vi "xboxToggle.vi"   [LabVIEW 2017]
uses:
  globalUtilities.vi
types:
  T1 = cluster{"button info":cluster{"button 1":bool, "button 2":bool, "button 3":bool, "button 4":bool, "button 5":bool, "button 6":bool, "button 7":bool, "button 8":bool, "button 9":bool, "button 10":bool, "button 11":bool, "button 12":bool, "button 13":bool, "button 14":bool, "button 15":bool, "button 16":bool, "button 17":bool, "button 18":bool, "button 19":bool, "button 20":bool, "button 21":bool, "button 22":bool, "button 23":bool, "button 24":bool, "button 25":bool, "button 26":bool, "button 27":bool, "button 28":bool, "button 29":bool, "button 30":bool, "button 31":bool, "button 32":bool}, "direction info":cluster{"pov 1":i32, "pov 2":i32, "pov 3":i32, "pov 4":i32}, "axis info":cluster{"X axis":i32, "Y axis":i32, "Z axis":i32, "X axis rotation":i32, "Y axis rotation":i32, "Z axis rotation":i32, "U axis":i32, "V axis":i32}}
  T2 = cluster{"button 1":bool, "button 2":bool, "button 3":bool, "button 4":bool, "button 5":bool, "button 6":bool, "button 7":bool, "button 8":bool, "button 9":bool, "button 10":bool, "button 11":bool, "button 12":bool, "button 13":bool, "button 14":bool, "button 15":bool, "button 16":bool, "button 17":bool, "button 18":bool, "button 19":bool, "button 20":bool, "button 21":bool, "button 22":bool, "button 23":bool, "button 24":bool, "button 25":bool, "button 26":bool, "button 27":bool, "button 28":bool, "button 29":bool, "button 30":bool, "button 31":bool, "button 32":bool}
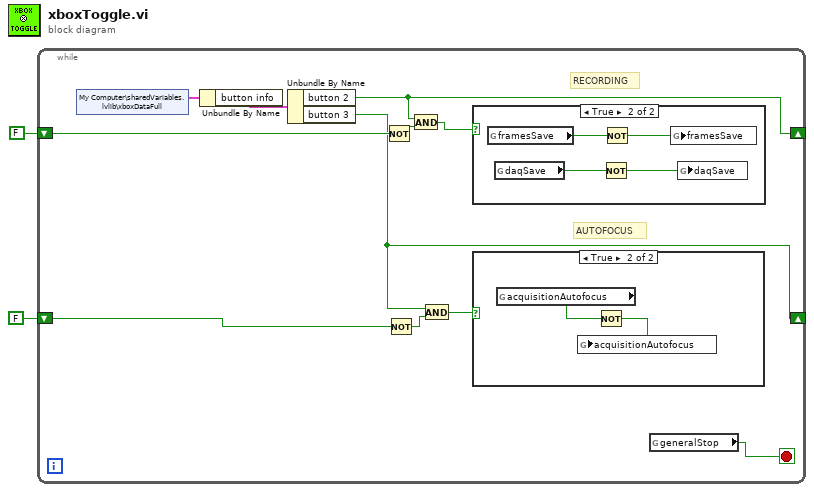
[diagram p0: block diagram]
diagram:
  n1 = while {
    shift-right: [w10] -> _
    shift-left: FALSE -> [w11]
    shift-right: [w3] -> _
    shift-left: FALSE -> [w6]
    stop <- w7 stop-if-true
    # "AUTOFOCUS"
    # "RECORDING"
    n2 = shared-variable "My Computer\\sharedVariables.lvlib\\xboxDataFull"() -> (w13:T1)  [unwired: 1 in, 1 out]
    n3 = Unbundle By Name(w13) -> ("button info"=w12:T2)
    n4 = Unbundle By Name(w12) -> ("button 2"=w10:bool, "button 3"=w3:bool)
    n5 = Not(x=w11) -> (.not. x?=w9:bool)
    n6 = Not(x=w6) -> (.not. x?=w5:bool)
    n7 = And(x=w10, y=w9) -> (x .and. y?=w8:bool)
    n8 = And(x=w3, y=w5) -> (x .and. y?=w4:bool)
    n9 = case shown="True" w8 {
      frame False {
      }
      frame True {
        n10 = global read "globalUtilities.vi" "framesSave"() -> (w19:bool)
        n11 = global read "globalUtilities.vi" "daqSave"() -> (w16:bool)
        n12 = Not(x=w16) -> (.not. x?=w17:bool)
        n13 = Not(x=w19) -> (.not. x?=w18:bool)
        n14 = global write "globalUtilities.vi" "framesSave"(w18) -> ()
        n15 = global write "globalUtilities.vi" "daqSave"(w17) -> ()
      }
    }
    n16 = case shown="True" w4 {
      frame False {
      }
      frame True {
        n17 = global read "globalUtilities.vi" "acquisitionAutofocus"() -> (w15:bool)
        n18 = Not(x=w15) -> (.not. x?=w14:bool)
        n19 = global write "globalUtilities.vi" "acquisitionAutofocus"(w14) -> ()
      }
    }
    n20 = global read "globalUtilities.vi" "generalStop"() -> (w7:bool)
  }
